vi "MakeFrameNumbers.vi"(9 "Array":dbl[](array[numeric]), 10 "Number of frames":i32) -> (2 "Frame Number Array":dbl[](array[numeric]))   [LabVIEW 2015]
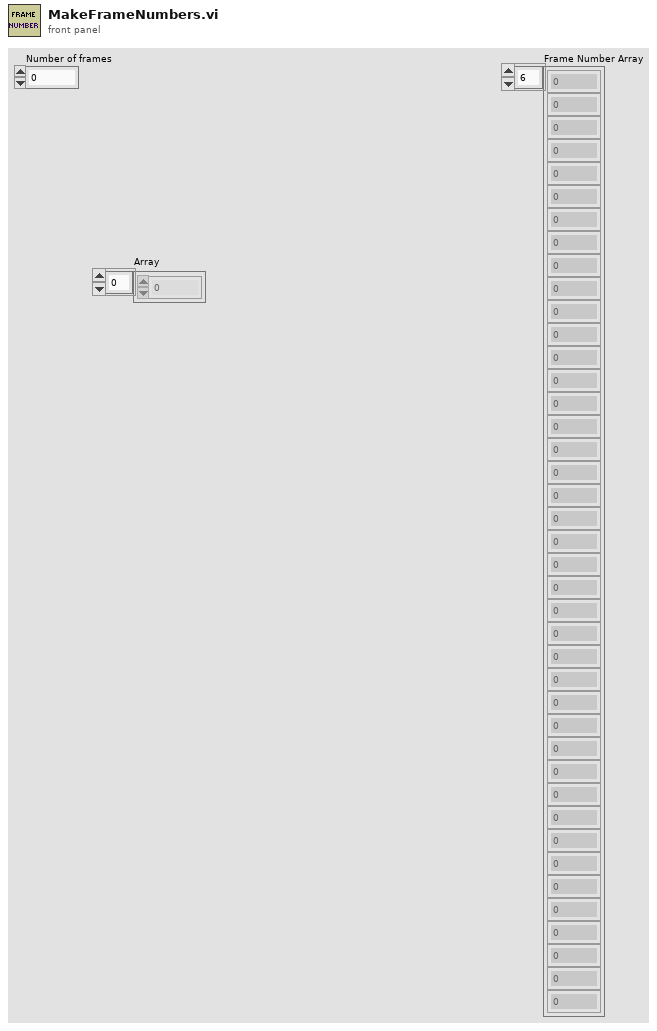
[diagram p1: front panel]
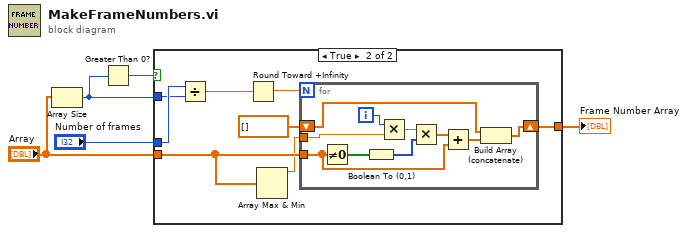
[diagram p0: block diagram]
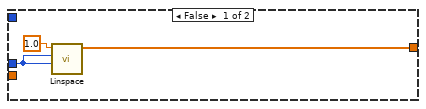
[diagram p2: hidden frame]
diagram:
  n1 = Array Size(array="Array") -> (size(s)=w3:i32)
  n2 = Greater Than 0?(x=w3) -> (x > 0?=w2:bool)
  n3 = case shown="True" w2 {
    tunnel: "Number of frames" -> [w7 w16]
    tunnel: w3 -> [_ w15]
    tunnel: "Array" -> [_ w10]
    tunnel: [w6 w12] -> w1
    frame False {
      n4 = call "Linspace.vi"("n"=w7, "End"=w7, "Start"=1.0) -> ("Array"=w6:dbl[])  [unwired: 8 in]
    }
    frame True {
      n5 = Divide(x=w16, y=w15) -> (x/y=w14:dbl)
      n6 = Round Toward +Infinity(x=w14) -> (ceil(x): smallest int >= x=w13:dbl)
      n7 = Array Max & Min(array=w10) -> (max value=w9:dbl)  [unwired: 3 out]
      n8 = for {
        N: w13 -> [_]
        tunnel: w10 -> [w18]
        shift-right: [w26] -> w12
        shift-left: dbl[] [] ("Array") -> [w19]
        tunnel: w9 -> [w17]
        i -> [w25]
        n9 = Not Equal To 0?(x=w18) -> (x != 0?=w23:bool[])
        n10 = Boolean To (0,1)(Boolean=w23) -> (0, 1=w21:i16[])
        n11 = Multiply(x=w25, y=w17) -> (x*y=w22:dbl)
        n12 = Multiply(x=w22, y=w21) -> (x*y=w20:dbl[])
        n13 = Add(x=w20, y=w18) -> (x+y=w24:dbl[])
        n14 = Build Array (concatenate)(w19, w24) -> (w26:dbl[])
      }
    }
  }
  "Frame Number Array" <- w1
